vi "Get_Trace (SubVI).vi"(6 "max points per trace (all)":i32=-1, 7 "database URL":path=path "\\\\HousesoftheHoly\\Default_Database", 8 "Filter?":bool, 10 "time interval":T2, 11 "Array in":string[](array[string])) -> (3 "Array out":T1(array[cluster]))   [LabVIEW 2020]
uses:
  <vilib>/lvdsc/historical/Read Trace (Numeric).vi
  <vilib>/lvdsc/NI_DSC.lvlib
  <vilib>/Analysis/NI_AALBase.lvlib
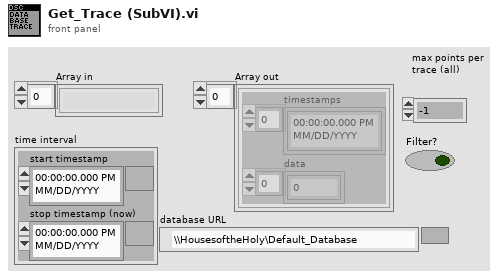
[diagram p1: front panel]
types:
  T1 = cluster{"timestamps":timestamp[], "data":dbl[]}[]
  T2 = cluster{"start timestamp":timestamp, "stop timestamp (now)":timestamp}
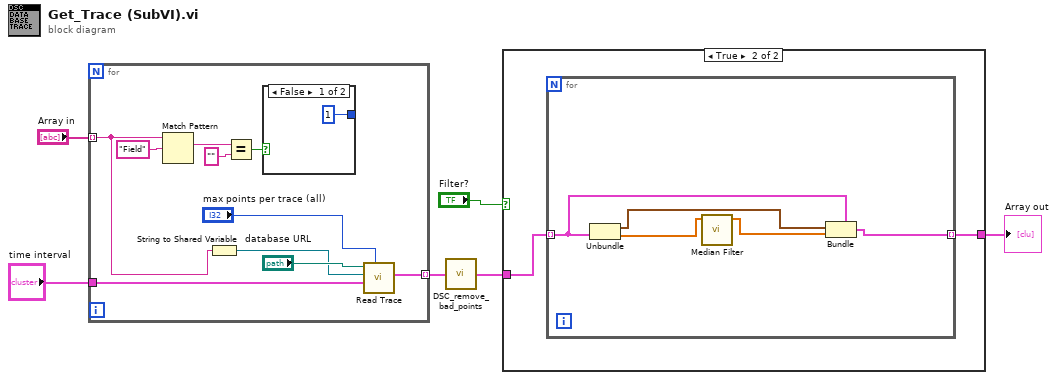
[diagram p0: block diagram]
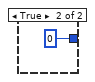
[diagram p3: hidden frame]
diagram:
  n1 = for {
    tunnel: "Array in" -> [w8] mode=indexing
    tunnel: [w10] -> w4 mode=indexing
    tunnel: "time interval" -> [w11]
    n2 = Match Pattern(string=w8, regular expression="Field") -> (match substring=w13:string)  [unwired: 1 in, 3 out]
    n3 = String to Shared Variable(0:w8) -> (2:w7:refnum<k21>)  [unwired: 1 out]
    n4 = Equal?(x=w13, y="") -> (x = y?=w14:bool)
    n5 = case shown="False" w14 {
      tunnel: [1 ("Active Y Scale") 0 ("Active Y Scale")] -> _
      frame False {
      }
      frame True {
      }
    }
    n6 = call-poly <vilib>:"Read Trace.vi"("max points per trace (all)"="max points per trace (all)", "time interval"=w11, "trace name"=w7, "database URL"="database URL") -> ("historical trace"=w10:cluster{"timestamps":timestamp[], "data":dbl[]})  [unwired: 4 in, 3 out]
  }
  n7 = call "DSC_remove_bad_points.vi"("Database Trace In"=w4) -> ("Database Trace Out"=w3:T1)
  n8 = case shown="True" "Filter?" {
    tunnel: w3 -> [w19 w21]
    tunnel: [w19 w20] -> w2
    frame False {
    }
    frame True {
      n9 = for {
        tunnel: w21 -> [w26] mode=indexing
        tunnel: [w22] -> w20 mode=indexing
        n10 = Unbundle(w26) -> ("timestamps"=w24:timestamp[], "data"=w25:dbl[])
        n11 = call <vilib>:"Median Filter.vi"("X"=w25) -> ("Filtered X"=w23:dbl[])  [unwired: 9 in, 1 out]
        n12 = Bundle(cluster=w26, "timestamps"=w24, "data"=w23) -> (w22:cluster{"timestamps":timestamp[], "data":dbl[]})
      }
    }
  }
  "Array out" <- w2
